vi "Call 2 Point Selection By Reference.vi"(7 "DisplayFilter":u8(ring)=7 items=["K_CHAN_R", "K_CHAN_W", "K_CHAN_RW", "K_CHAN_VOLT", "K_CHAN_FAULT", "K_ALL", "K_CUSTOM", "K_CHAN_R_VIS", "K_CHAN_W_VIS", "K_CHAN_RW_VIS", "K_CHAN_VOLT_VIS", "K_CHAN_FAULT_VIS"], 8 "error in (no error)":errorcluster, 9 "NIVS.System Definition Root":refnum<k24>, 10 "NodePaths":string[](array[string])) -> (0 "error out":errorcluster, 2 "Selected NodePaths":string[](array[string]))   [LabVIEW 2011]
uses:
  NationalInstruments.VeriStand.SystemStorage
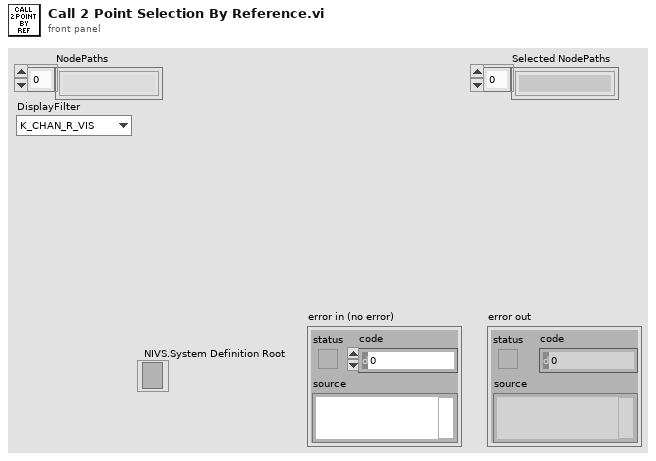
[diagram p1: front panel]
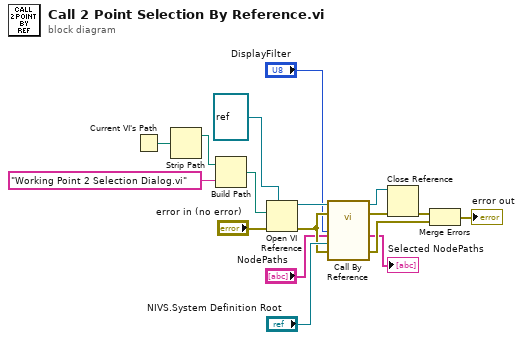
[diagram p0: block diagram]
diagram:
  n1 = Current VI's Path() -> (path=w17:path)
  n2 = Strip Path(path=w17) -> (stripped path=w5:path)  [unwired: 1 out]
  n3 = Build Path(base path=w5, name or relative path="Working Point 2 Selection Dialog.vi") -> (appended path=w15:path)
  n4 = Open VI Reference(type specifier VI Refnum (for type only)=refnum<vi> refnum, vi path=w15, error in (no error)="error in (no error)") -> (vi reference=w13:refnum<vi>, error out=w11:errorcluster)  [unwired: 3 in]
  n5 = call-by-ref "?"(reference=w13, error in=w11, "DisplayFilter"="DisplayFilter", 8:"error in (no error)"=w11, "NIVS.System Definition Root"="NIVS.System Definition Root", "NodePaths"="NodePaths") -> (reference out=w8:refnum<vi>, error out=w7:errorcluster, 0:"error out"=w10:errorcluster, "Selected NodePaths"=→"Selected NodePaths":string[])  [unwired: 6 in]
  n6 = Close Reference(reference=w8, error in (no error)=w7) -> (error out=w6:errorcluster)
  n7 = Merge Errors(w6, w10) -> (→"error out":errorcluster)
